vi "LSCI332 SetRamp.vi"(0 "VISA Rsrc":refnum<visa-resource-name>="GPIB0::12::INSTR", 5 "Boucle(1)":u32(ring) caption="Boucle" items=["Boucle 1", "Boucle 2"], 7 "RampPar":cluster{"Rampe Activée":bool, "RateVal":dbl}={"Rampe Activée"=FALSE, "RateVal"=0.1} caption="Paramètres de Rampe" {"RateVal" min=0.1 max=100.0 step=0.1}, 11 "error in (no error)":errorcluster) -> (15 "error out":errorcluster)   [LabVIEW 2019]
doc: "Ce VI écrit les paramètres limites de contrôle dans le contrôleur."
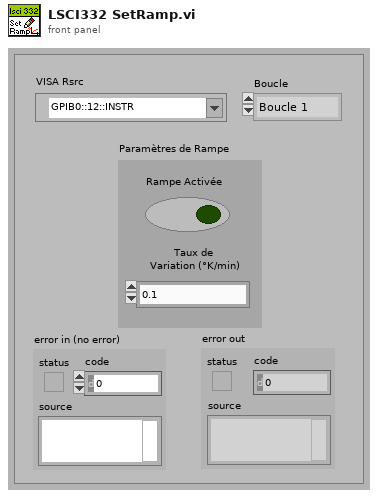
[diagram p1: front panel]
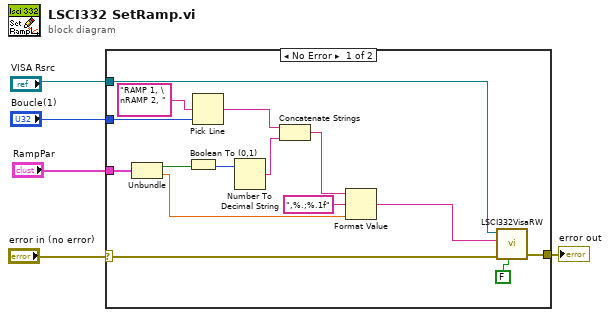
[diagram p0: block diagram]
diagram:
  n1 = case shown="No Error" "error in (no error)" {
    selector: "error in (no error)" -> [w18 w21]
    tunnel: "VISA Rsrc" -> [w20 _]
    tunnel: "Boucle(1)" -> [w15 _]
    tunnel: [w19 w21] -> w3
    tunnel: "RampPar" -> [w8 _]
    frame No Error {
      n2 = Unbundle(w8) -> ("Rampe Activée"=w7:bool, "RateVal"=w6:dbl)
      n3 = Boolean To (0,1)(Boolean=w7) -> (0, 1=w12:i16)
      n4 = Pick Line(multi-line string="RAMP 1, \nRAMP 2, ", line index=w15) -> (output string=w14:string)  [unwired: 1 in]
      n5 = Number To Decimal String(number=w12) -> (decimal integer string=w13:string)  [unwired: 1 in]
      n6 = Concatenate Strings(w14, w13) -> (w11:string)
      n7 = Format Value(string ("")=w11, format string=",%.;%.1f", value (0)=w6) -> (output string=w9:string)
      n8 = call <userlib>:"LSCI332VisaRW.vi"("Lecture?(T)"=FALSE, "error in (no error)"=w18, "ChaineCom"=w9, "VISA Rsrc"=w20) -> ("error out"=w19:errorcluster)  [unwired: 3 in, 3 out]
    }
    frame Error {
    }
  }
  "error out" <- w3
